vi "skelett_4.3_2020.vi"() -> ()   [LabVIEW 2017]
panel:
  in  "Registerkarte":enum32{"Berechnung", "Debug"}(tab)
  out "2D이미지 2":T1(plugin-control) caption="2D Grab 이미지"
  out "2D이미지":T1(plugin-control) caption="2D Grab 이미지"
  in  "Objekt":T2(ring)=enum."Text"
  in  "invert input":enum16{"invert", "bypass"}(ring)=enum."bypass"
  out "Input":i16[][](graph)
  out "Output":dbl[][](graph)
  out "While \nIterationen":i32
  in  "Modus":enum16{"thinning", "skeleton"}(ring)
  in  "y":bool
  out "0, 1":u8[][](array[numeric])
  out "배열":bool[][](array[boolean])
  out "Numerisch (Ausgang)":i32
  in  "[user-specified font]":T3={"Font Name:"="test", "Size"=70, "Strikeout?"=FALSE, "Italic?"=TRUE, "Underline?"=FALSE, "Outline?"=FALSE, "Shadow?"=FALSE, "Bold?"=TRUE} caption="[Benutzerdefinierte Schriftart]"
  in  "text orientation":T4(ring) caption="Textausrichtung"
  in  "text":string="4   56\ngg" caption="Text"
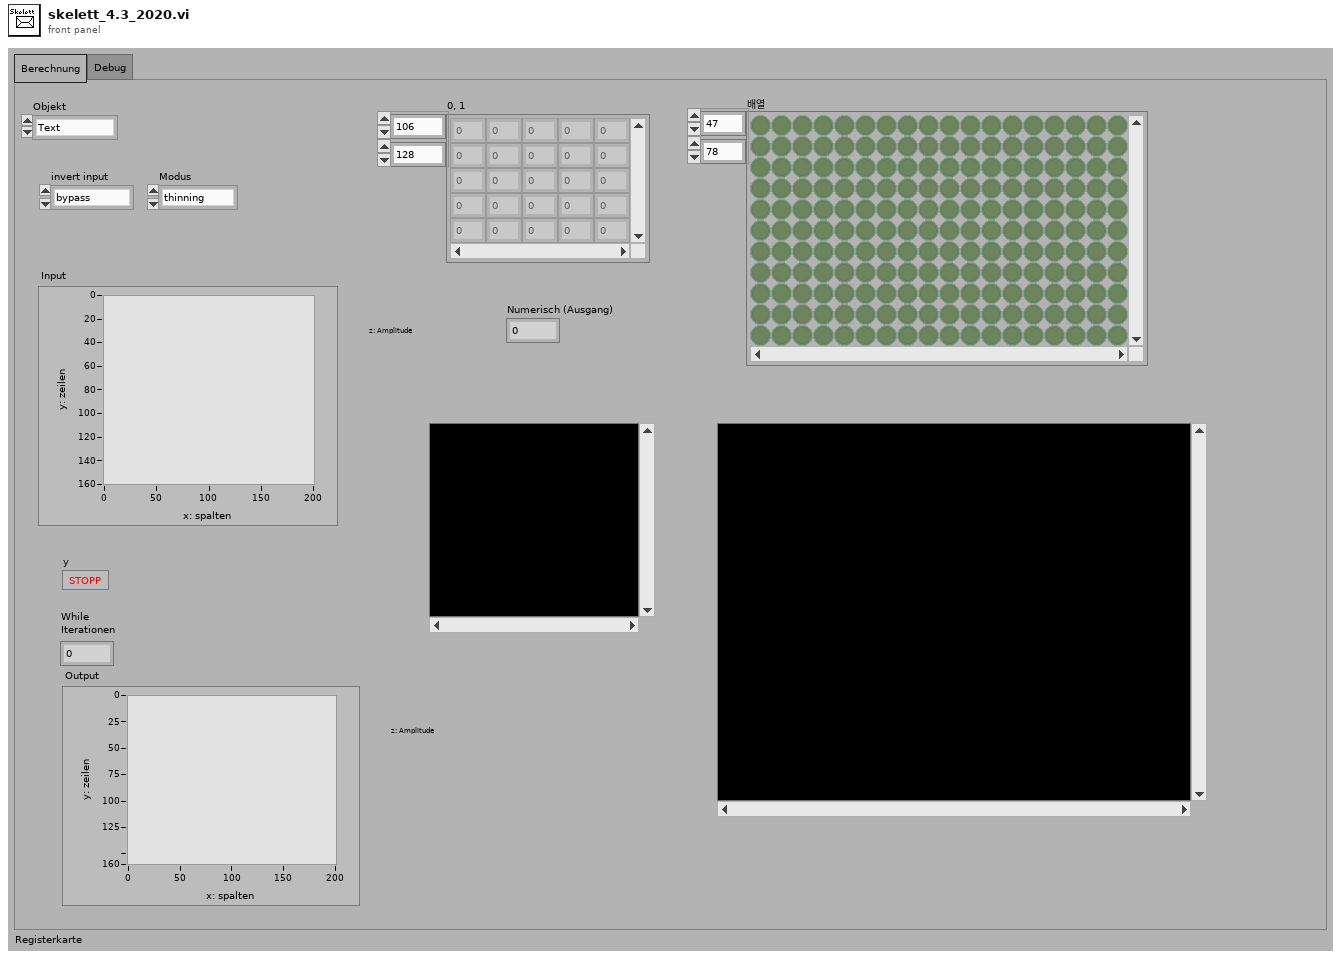
[diagram p1: front panel]
types:
  T1 = typedef "IMAQ Image.ctl" = refnum<image>
  T2 = enum16{"Rechteck", "Ellipse", "Oval", "Kreis", "Text"}
  T3 = cluster{"Font Name:":string, "Size":i16, "Strikeout?":bool, "Italic?":bool, "Underline?":bool, "Outline?":bool, "Shadow?":bool, "Bold?":bool}
  T4 = enum16{"None", "Stacked", "Clockwise", "Counterclockwise"}
  T5 = typedef "Image Type" = u32
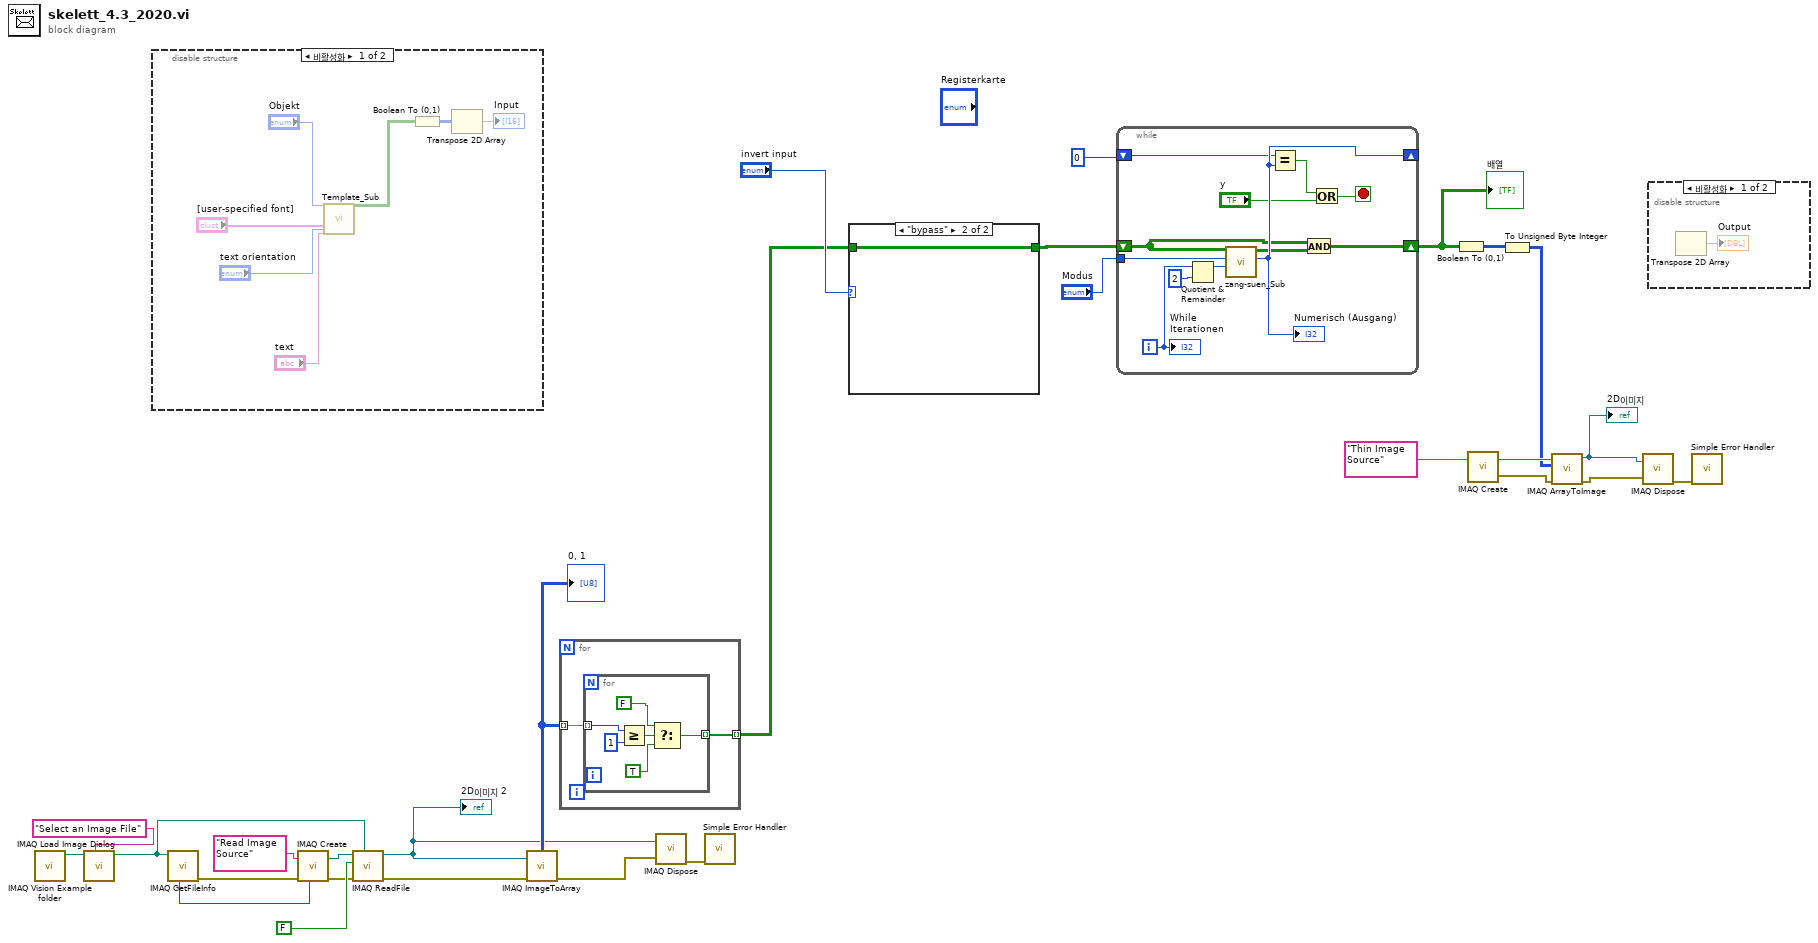
[diagram p0: block diagram]
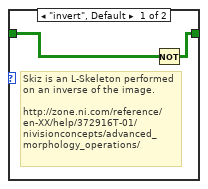
[diagram p4: hidden frame]
diagram:
  n1 = call "IMAQ Vision Example folder.vi"() -> ("Example Image Path"=w6:path)  [unwired: 11 in]
  n2 = call "IMAQ Load Image Dialog"("Prompt"="Select an Image File" ("prompt"), "Start Path"=w6) -> ("Path"=w10:path)  [unwired: 7 in, 2 out]
  n3 = disable-structure shown="비활성화" {
    frame Disabled {
      n4 = call "Template_Sub.vi"("Objekt"="Objekt", "[user-specified font]"="[user-specified font]", "text orientation"="text orientation", "text"="text") -> ("Template"=w29:bool[][])  [unwired: 23 in]
      n5 = Boolean To (0,1)(Boolean=w29) -> (0, 1=w34:i16[][])
      n6 = Transpose 2D Array(2D array=w34) -> (transposed array=→"Input":i16[][])
    }
    frame Enabled {
    }
  }
  n7 = call "IMAQ GetFileInfo"("File Path"=w10) -> ("error out"=w8:errorcluster, "Image Type"=w7:T5)  [unwired: 4 in, 5 out]
  n8 = call "IMAQ Create"("Image Name"="Read Image Source", "Image Type"=w7, "error in (no error)"=w8) -> ("New Image"=w5:T1, "error out"=w4:errorcluster)  [unwired: 2 in]
  n9 = call "IMAQ ReadFile"("File Path"=w10, "error in (no error)"=w4, "Load Color Palette? (No)"=FALSE, "Image"=w5) -> ("error out"=w13:errorcluster, "Image Out"=w15:T1)  [unwired: 3 in, 3 out]
  "2D이미지 2" <- w15
  n10 = call "IMAQ ImageToArray"("error in (no error)"=w13, "Image"=w15) -> ("error out"=w14:errorcluster, "Image Pixels (U8)"=w16:u8[][])  [unwired: 2 in, 3 out]
  "0, 1" <- w16
  n11 = for {
    tunnel: w16 -> [w37] mode=indexing
    tunnel: [w36] -> w2 mode=indexing
    n12 = for {
      tunnel: w37 -> [w41] mode=indexing
      tunnel: [w40] -> w36 mode=indexing
      n13 = Greater Or Equal?(x=w41, y=u8 1) -> (x >= y?=w43:bool)
      n14 = Select(t=FALSE, s=w43, f=TRUE) -> (s? t:f=w40:bool)
    }
  }
  n15 = call "IMAQ Dispose"("Image"=w15, "error in (no error)"=w14) -> ("error out"=w11:errorcluster)  [unwired: 4 in]
  n16 = call <vilib>:"Simple Error Handler.vi"("error in (no error)"=w11) -> ()  [unwired: 4 in, 5 out]
  n17 = case shown="\"bypass\"" "invert input" {
    tunnel: w2 -> [w45 w46]
    tunnel: [w44 w46] -> w17
    frame "invert", Default {
      # "Skiz is an L-Skeleton performed on an inverse of the image.\n\nhttp://zone.ni.com/reference/en-XX/help/372916T-01/nivisionconcepts/advanced_morphology_operations/"
      n18 = Not(x=w45) -> (.not. x?=w44:bool[][])
    }
    frame "bypass" {
    }
  }
  n19 = while {
    shift-right: [w55] -> w1
    shift-left: w17 -> [w47]
    shift-right: [w54] -> _
    shift-left: 0 -> [w53]
    tunnel: "Modus" -> [w52]
    i -> [w58]
    stop <- w50 stop-if-true
    n20 = Quotient & Remainder(x=w58, y=2) -> (x-y*floor(x/y)=w56:i32)  [unwired: 1 out]
    n21 = call "zang-suen_Sub.vi"("Numerisch (Eingang)"=w56, "Modus"=w52, "Template"=w47) -> ("Numerisch (Ausgang)"=w54:i32, "Array"=w48:bool[][])  [unwired: 7 in]
    "Numerisch (Ausgang)" <- w54
    n22 = Equal?(x=w53, y=w54) -> (x = y?=w51:bool)
    n23 = And(x=w47, y=w48) -> (x .and. y?=w55:bool[][])
    n24 = Or(x=w51, y="y") -> (x .or. y?=w50:bool)
    "While \nIterationen" <- w58
  }
  "배열" <- w1
  n25 = Boolean To (0,1)(Boolean=w1) -> (0, 1=w19:i16[][])
  n26 = call "IMAQ Create"("Image Name"="Thin Image Source") -> ("New Image"=w24:T1, "error out"=w25:errorcluster)  [unwired: 4 in]
  n27 = To Unsigned Byte Integer(number=w19) -> (unsigned 8bit integer=w18:u8[][])
  n28 = call "IMAQ ArrayToImage"("error in (no error)"=w25, "Image Pixels (U8)"=w18, "Image"=w24) -> ("error out"=w21:errorcluster, "Image Out"=w22:T1)  [unwired: 7 in]
  "2D이미지" <- w22
  n29 = call "IMAQ Dispose"("Image"=w22, "error in (no error)"=w21) -> ("error out"=w23:errorcluster)  [unwired: 4 in]
  n30 = disable-structure shown="비활성화" {
    frame Disabled {
      n31 = Transpose 2D Array() -> (transposed array=→"Output":dbl[][])  [unwired: 1 in]
    }
    frame Enabled {
    }
  }
  n32 = call <vilib>:"Simple Error Handler.vi"("error in (no error)"=w23) -> ()  [unwired: 4 in, 5 out]
